vi "Module Cleanup.vi"(8 "error in (no error)":errorcluster, 11 "GUI Manager Module in":refnum<class "GUI Manager Module.lvclass">) -> (0 "error out":errorcluster, 3 "GUI Manager Module out":refnum<class "GUI Manager Module.lvclass">)   [LabVIEW 2020, in "VolatusGUI.lvlib" / "GUI Manager Module.lvclass"]
uses:
  GUI Manager Module.lvclass
  GUI Manager Module.lvclass/GUI Manager Module.ctl
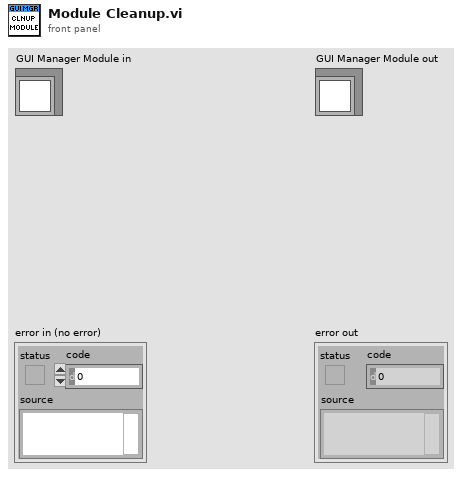
[diagram p1: front panel]
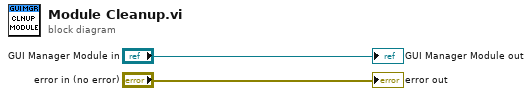
[diagram p0: block diagram]
diagram:
  "error out" <- "error in (no error)"
  "GUI Manager Module out" <- "GUI Manager Module in"
